vi "Move.vi"(8 "error in (no error)":errorcluster, 9 "New path":string, 10 "Path":string, 11 "FTP in":refnum<class "FTP.lvclass">) -> (0 "error out":errorcluster, 3 "FTP out":refnum<class "FTP.lvclass">)   [LabVIEW 2015, in "RT Management.lvlib" / "FTP.lvclass"]
uses:
  FTP.lvclass
  FTP.lvclass/FTP.ctl
  Get Session.vi
  <vilib>/Utility/error.llb/Trim Whitespace.vi
  File Transfer Behavior/File Transfer Behavior.lvclass
  <vilib>/FTP/NI_FTP.lvlib
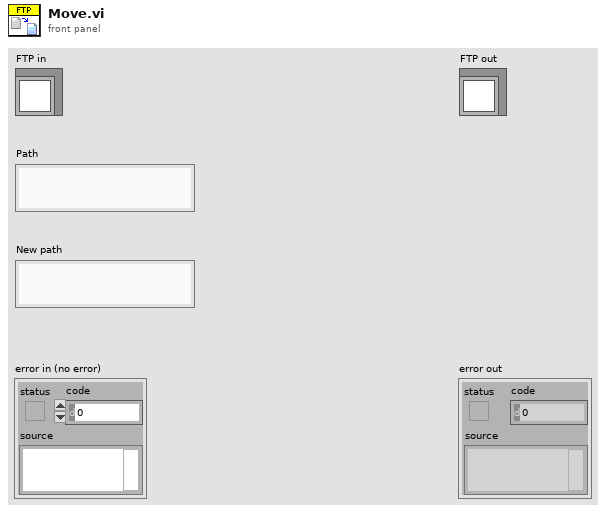
[diagram p1: front panel]
types:
  T1 = typedef "NI_FTP.lvlib/FTP Session.ctl" = refnum<k5>
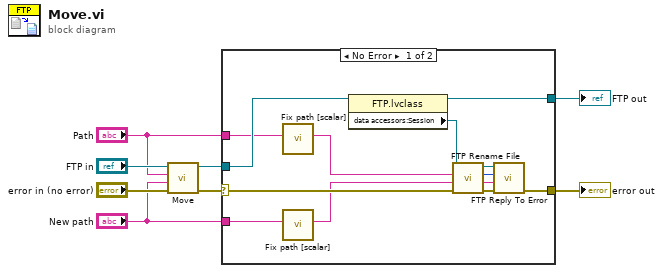
[diagram p0: block diagram]
diagram:
  n1 = call-parent "Move.vi"("error in (no error)"="error in (no error)", "New path"="New path", "Path"="Path", "File Transfer Behavior in"="FTP in") -> ("error out"=w5:errorcluster, "File Transfer Behavior out"=w3:refnum<class "FTP.lvclass">)  [unwired: 6 in]
  n2 = case shown="No Error" w5 {
    selector: w5 -> [w20 w23]
    tunnel: [w18 w23] -> w8
    tunnel: w3 -> [w21 w22]
    tunnel: [w19 w22] -> w7
    tunnel: "New path" -> [w9 _]
    tunnel: "Path" -> [w10 _]
    frame No Error {
      n3 = call "Fix path [scalar].vi"("Path in"=w10) -> ("Path out"=w16:string)  [unwired: 8 in, 2 out]
      n4 = call "Fix path [scalar].vi"("Path in"=w9) -> ("Path out"=w11:string)  [unwired: 8 in, 2 out]
      n5 = property class="FTP.lvclass"(reference=w21) -> (reference out=w19:refnum<class "FTP.lvclass">, "data accessors:Session"=w17:T1)  [unwired: 1 in, 1 out]
      n6 = call <vilib>:"FTP Rename File.vi"("error in (no error)"=w20, "new name"=w11, "old name"=w16, "ftp session"=w17) -> ("error out"=w15:errorcluster, "reply string"=w14:string, "reply code"=w13:i32, "ftp session out"=w12:T1)  [unwired: 4 in]
      n7 = call <vilib>:"FTP Reply To Error.vi"("error in (no error)"=w15, "reply string in"=w14, "reply code in"=w13, "ftp session"=w12) -> ("error out"=w18:errorcluster)  [unwired: 3 out]
    }
    frame Error {
    }
  }
  "error out" <- w8
  "FTP out" <- w7
